vi "校准时间.vi"() -> ()   [LabVIEW 2020]
panel:
  out "时间差":dbl
  out "计算机时间":string
  out "源表时间":string
  out "日期/时间字符串":string
  in  "校准时间":bool
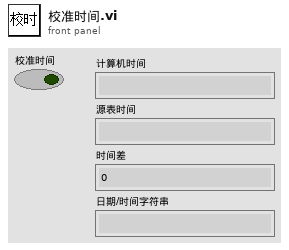
[diagram p1: front panel]
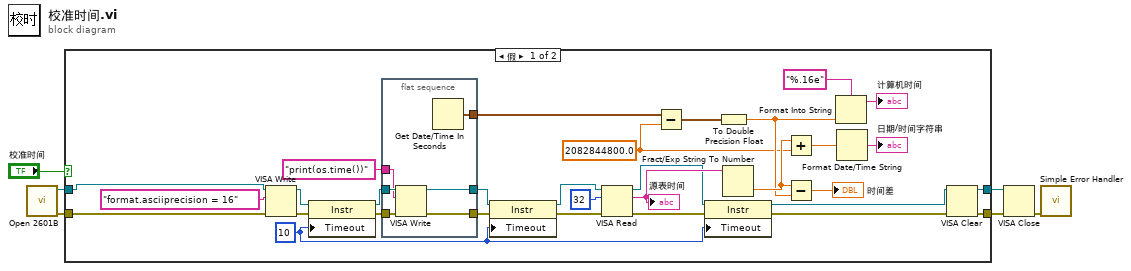
[diagram p0: block diagram]
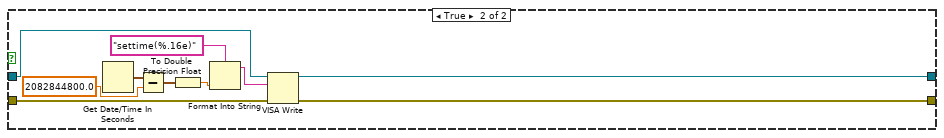
[diagram p2: hidden frame]
diagram:
  n1 = call "Open 2601B.vi"() -> ("错误输出"=w4:errorcluster, "VISA资源名称输出"=w5:refnum<visa-resource-name>)  [unwired: 10 in]
  n2 = case shown="假" "校准时间" {
    tunnel: w4 -> [w9 w53]
    tunnel: w5 -> [w10 w52]
    tunnel: [w7 w51] -> w2
    tunnel: [w8 w50] -> w3
    frame False {
      w13 = u32 10 ("General Settings:Timeout Value")
      w14 = 2082844800.0 ("x-y")
      n3 = VISA Write(VISA resource name=w10, write buffer="format.asciiprecision = 16" ("格式字符串"), error in (no error)=w9) -> (VISA resource name out=w18:refnum<visa-resource-name>, error out=w19:errorcluster)  [unwired: 1 out]
      n4 = property class="Instr"(reference=w18, error in=w19, "Timeout"=w13) -> (reference out=w28:refnum<visa-resource-name>, error out=w29:errorcluster)
      n5 = flat-sequence {
        tunnel: [w43] -> w20
        tunnel: [w42] -> w21
        tunnel: w28 -> [w41]
        tunnel: w29 -> [w40]
        tunnel: "print(os.time())" ("写入缓冲区") -> [w39]
        tunnel: [w38] -> w31
        frame #0 {
          n6 = VISA Write(VISA resource name=w41, write buffer=w39, error in (no error)=w40) -> (VISA resource name out=w43:refnum<visa-resource-name>, error out=w42:errorcluster)  [unwired: 1 out]
          n7 = Get Date/Time In Seconds() -> (seconds since 1Jan1904=w38:timestamp)
        }
      }
      n8 = property class="Instr"(reference=w20, error in=w21, "Timeout"=w13) -> (reference out=w23:refnum<visa-resource-name>, error out=w22:errorcluster)
      n9 = VISA Read(VISA resource name=w23, byte count=u32 32 ("字节总数"), error in (no error)=w22) -> (VISA resource name out=w24:refnum<visa-resource-name>, read buffer=w30:string, error out=w25:errorcluster)  [unwired: 1 out]
      "源表时间" <- w30
      n10 = Subtract(x=w31, y=w14) -> (x-y=w32:timestamp)
      n11 = property class="Instr"(reference=w24, error in=w25, "Timeout"=w13) -> (reference out=w26:refnum<visa-resource-name>, error out=w27:errorcluster)
      n12 = To Double Precision Float(number=w32) -> (double precision float=w34:dbl)
      n13 = Fract/Exp String To Number(string=w30) -> (number=w35:dbl)  [unwired: 3 in, 1 out]
      n14 = Add(x=w35, y=w14) -> (x+y=w33:dbl)
      n15 = Subtract(x=w35, y=w34) -> (x-y=→"时间差":dbl)
      n16 = Format Into String(format string="%.16e" ("格式字符串"), w34) -> (resulting string=→"计算机时间":string)  [unwired: 2 in, 1 out]
      n17 = Format Date/Time String(seconds (now)=w33) -> (date/time string=→"日期/时间字符串":string)  [unwired: 2 in]
      n18 = VISA Clear(VISA resource name=w26, error in (no error)=w27) -> (VISA resource name out=w8:refnum<visa-resource-name>, error out=w7:errorcluster)
    }
    frame True {
      n19 = Get Date/Time In Seconds() -> (seconds since 1Jan1904=w47:timestamp)
      n20 = Subtract(x=w47, y=2082844800.0 ("x-y")) -> (x-y=w48:timestamp)
      n21 = To Double Precision Float(number=w48) -> (double precision float=w49:dbl)
      n22 = Format Into String(format string="settime(%.16e)" ("格式字符串"), w49) -> (resulting string=w44:string)  [unwired: 2 in, 1 out]
      n23 = VISA Write(VISA resource name=w52, write buffer=w44, error in (no error)=w53) -> (VISA resource name out=w50:refnum<visa-resource-name>, error out=w51:errorcluster)  [unwired: 1 out]
    }
  }
  n24 = VISA Close(VISA resource name=w3, error in (no error)=w2) -> (error out=w1:errorcluster)
  n25 = call <vilib>:"Simple Error Handler.vi"("error in (no error)"=w1) -> ()  [unwired: 4 in, 5 out]
